vi "Write MODBUS resource name.vi"(8 "error in (no error)":errorcluster, 10 "MODBUS resource name":refnum<visa-resource-name>="485", 11 "MODBUS in":refnum<class "MODBUS.lvclass">) -> (0 "error out":errorcluster, 3 "MODBUS out":refnum<class "MODBUS.lvclass">)   [LabVIEW 2016, in "MODBUS.lvclass"]
uses:
  MODBUS.lvclass
  MODBUS.lvclass/MODBUS.ctl
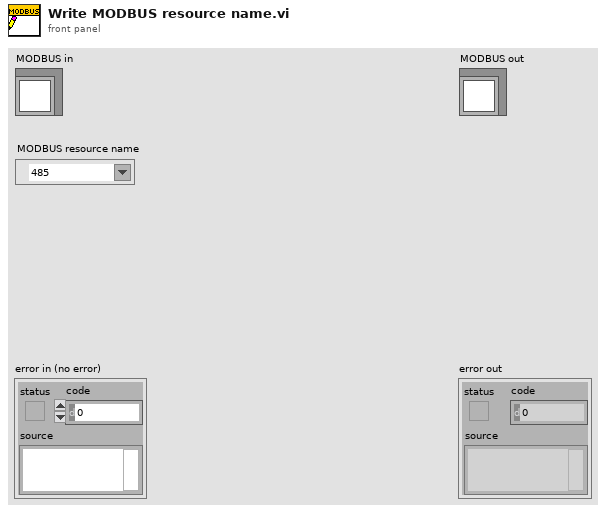
[diagram p1: front panel]
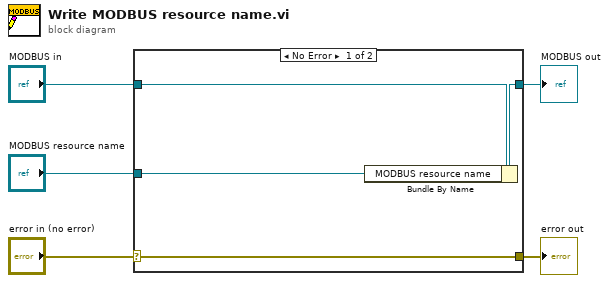
[diagram p0: block diagram]
diagram:
  n1 = case shown="No Error" "error in (no error)" {
    selector: "error in (no error)" -> [w9 w10]
    tunnel: [w9 w10] -> w4
    tunnel: [w7 w11] -> w2
    tunnel: "MODBUS in" -> [w8 w11]
    tunnel: "MODBUS resource name" -> [w6 _]
    frame No Error {
      n2 = Bundle By Name(cluster=w8, "MODBUS resource name"=w6) -> (w7:refnum<class "MODBUS.lvclass">)
    }
    frame Error {
    }
  }
  "error out" <- w4
  "MODBUS out" <- w2
